vi "Decode32bitTicRead.vi"(10 "ReadHex":string="This is simulation mode") -> (2 "Value":i32)   [LabVIEW 2018]
panel:
  out "Length(Bytes)":i32
  out "8bitBytes":bool[][](array[boolean])
  out "7bitBytes":bool[][](array[boolean])
  # "Decodes Pololu 32-bit Read Responses. Adapts to regular 4-byte, 8-bit replies, or 5-byte, 7-bit replies.\n\n\"To make sure that responses from one Tic do not get interpreted as a command for the other Tics, we have added a firmware feature for converting our normal serial responses (as described in the user's guide) from arbitrary binary data to 7-bit binary data before the response gets sent.  This feature is turned on by default, but you can also control it with a checkbox in the GUI software that we will be sending you later.\n\nHere's how the feature works: if you try to read some data from the Tic, the firmware generates the normal response as described in the user's guide, which can be arbitrary binary data.  Then, it shortens the response to be at most 7 bytes.  Then it adds a new byte to the response, which will contains the MSbs from the other bytes.  So it clears the MSbs in all the bytes of response, and puts the MSb values into that last byte.  The least-significant bit of the last byte corresponds to the MSb of the first response byte. \" -Jan Malasek, 20-May-2018"
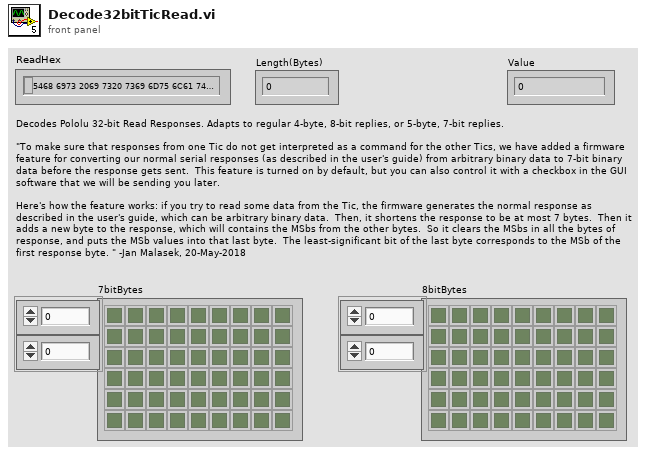
[diagram p1: front panel]
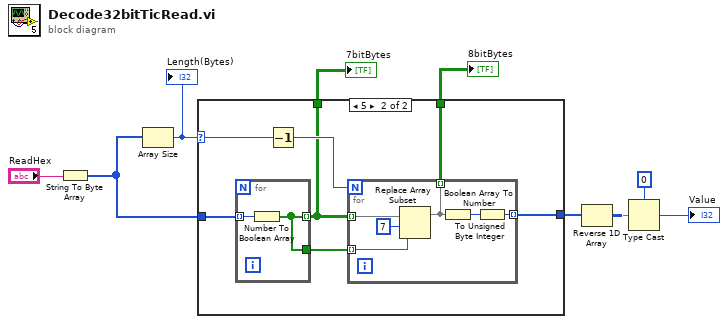
[diagram p0: block diagram]
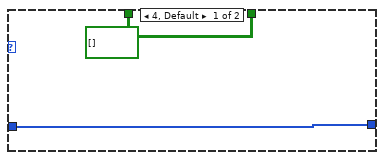
[diagram p2: hidden frame]
diagram:
  n1 = String To Byte Array(string="ReadHex") -> (unsigned byte array=w6:u8[])
  n2 = Array Size(array=w6) -> (size(s)=w5:i32)
  "Length(Bytes)" <- w5
  n3 = case shown="5" w5 {
    selector: w5 -> [_ w15]
    tunnel: w6 -> [w11 w17]
    tunnel: [w11 w14] -> w4
    tunnel: [w10 w13] -> w2
    tunnel: [w10 w12] -> w1
    frame 4, Default {
      w10 = bool[][] [] ("Boolean array")
    }
    frame 5 {
      n4 = for {
        tunnel: w17 -> [w26] mode=indexing
        tunnel: [w25] -> w13 mode=indexing
        tunnel: [w25] -> w18
        n5 = Number To Boolean Array(number=w26) -> (Boolean array=w25:bool[])
      }
      n6 = Decrement(x=w15) -> (x-1=w16:i32)
      n7 = for {
        N: w16 -> [_]
        tunnel: w13 -> [w24] mode=indexing
        tunnel: w18 -> [w23] mode=indexing
        tunnel: [w19] -> w14 mode=indexing
        tunnel: [w20] -> w12 mode=indexing
        n8 = Replace Array Subset(array=w24, new element=w23, index=7) -> (w20:bool[])
        n9 = Boolean Array To Number(Boolean array=w20) -> (number=w21:u32)
        n10 = To Unsigned Byte Integer(number=w21) -> (unsigned 8bit integer=w19:u8)
      }
    }
  }
  "7bitBytes" <- w2
  "8bitBytes" <- w1
  n11 = Reverse 1D Array(array=w4) -> (reversed array=w3:u8[])
  n12 = Type Cast(type=0, x=w3) -> (*(type *) &x=→"Value":i32)
